vi "Clock Array to Clock Map.vi"(8 "error in (no error)":errorcluster, 10 "Clock Conversion Array":T3[](array[typedef]), 11 "Clock Convert Map in":T1) -> (0 "error out":errorcluster, 3 "Clock Convert Map out":T1)   [LabVIEW 2021, in "Time_CIF_U.lvlib"]
uses:
  Time_CIF_U.lvlib
  Typedef/Clock Conversion Map.ctl
  Typedef/Timestamp Pair.ctl
  Typedef/Clock Conversion.ctl
  <vilib>/Utility/miscctls.llb/LVMapReplaceAction.ctl
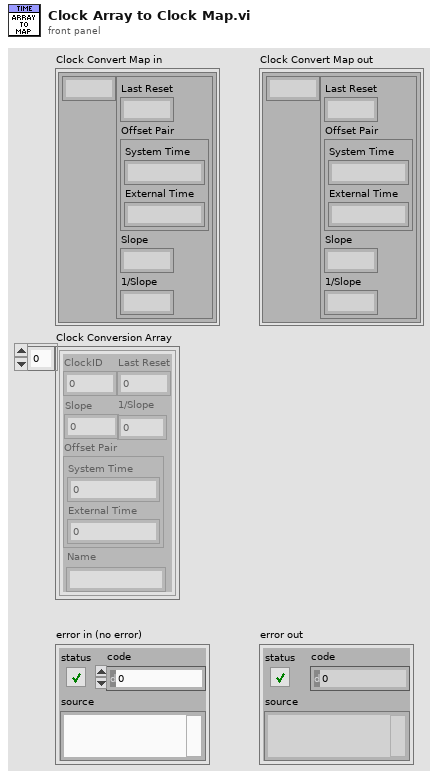
[diagram p1: front panel]
types:
  T1 = typedef "Time_CIF_U.lvlib/Clock Conversion Map.ctl" = map{u8, cluster{"Last Reset":i64, "Offset Pair":T2, "Slope":dbl, "1/Slope":dbl}}
  T2 = typedef "Time_CIF_U.lvlib/Timestamp Pair.ctl" = cluster{"System Time":i64, "External Time":i64}
  T3 = typedef "Time_CIF_U.lvlib/Clock Conversion.ctl" = cluster{"ClockID":u8, "Last Reset":i64, "Offset Pair":T2, "Slope":dbl, "1/Slope":dbl, "Name":string}
  T4 = typedef "LVMapReplaceAction.ctl" = enum32{"Modify Entry only if found", "Add or Modify Entry", "Delete Entry"}
  T5 = cluster{"Last Reset":i64, "Offset Pair":T2, "Slope":dbl, "1/Slope":dbl}
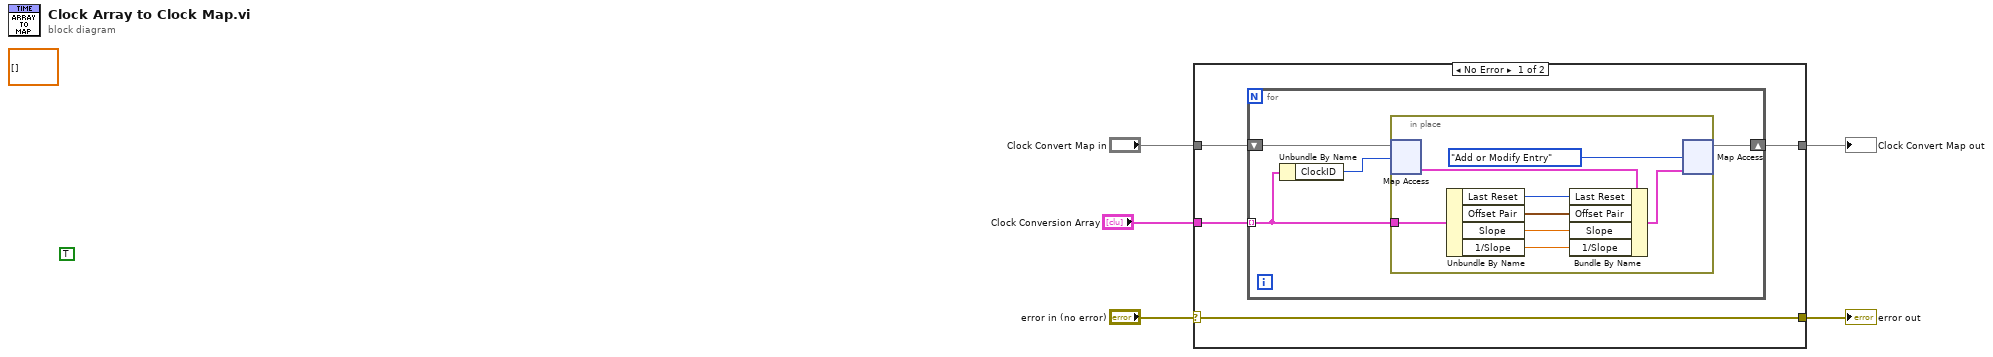
[diagram p0: block diagram]
diagram:
  (unwired) TRUE
  (unwired) dbl[][] []
  n1 = case shown="No Error" "error in (no error)" {
    selector: "error in (no error)" -> [w9 w23]
    tunnel: "Clock Convert Map in" -> [w8 w22]
    tunnel: [w9 w23] -> w3
    tunnel: "Clock Conversion Array" -> [w7 _]
    tunnel: [w6 w22] -> w1
    frame No Error {
      n2 = for {
        shift-right: [w10] -> w6
        shift-left: w8 -> [w13]
        tunnel: w7 -> [w11] mode=indexing
        n3 = Unbundle By Name(w11) -> ("ClockID"=w12:u8)
        n4 = in-place {
          in-place-border: w11 -> [w20]
          n5 = in-place-map #1(w13, w12) -> (w21:T5)  [unwired: 1 in, 1 out]
          n6 = Unbundle By Name(w20) -> ("Last Reset"=w19:i64, "Offset Pair"=w18:T2, "Slope"=w17:dbl, "1/Slope"=w14:dbl)
          n7 = Bundle By Name(cluster=w21, "Last Reset"=w19, "Offset Pair"=w18, "Slope"=w17, "1/Slope"=w14) -> (w16:T5)
          n8 = in-place-map #1(w16, LVMapReplaceAction."Add or Modify Entry" ("action")) -> (w10:T1)  [unwired: 2 out]
        }
      }
    }
    frame Error {
    }
  }
  "error out" <- w3
  "Clock Convert Map out" <- w1
